vi "DropDetection NaamaVision.vi"(8 "error in":errorcluster, 10 "Minimum Match Score":sgl=400.0, 11 "Path":path=path "Z:/Downloads/Fridge Pictures/1") -> (0 "error out":errorcluster, 1 "Number of Matches":i32, 2 "Matches (pixel)":T1(array[cluster]), 3 "Image Out":T2(plugin-control))   [LabVIEW 2013]
uses:
  <vilib>/vision/NI_Vision_Development_Module.lvlib
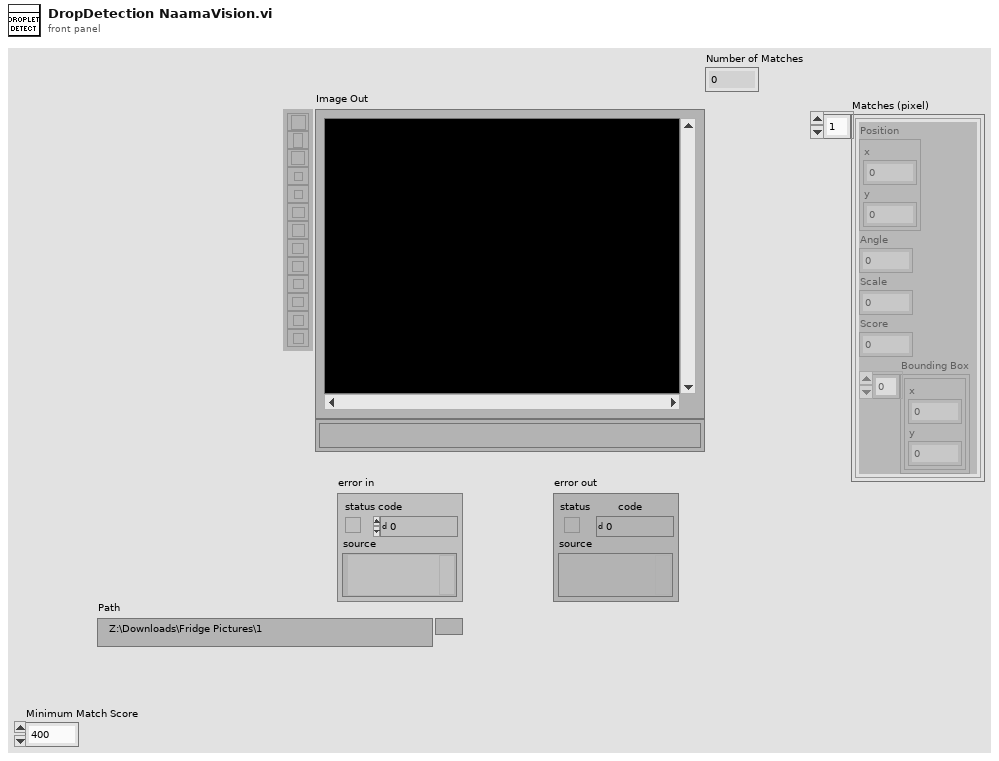
[diagram p1: front panel]
types:
  T1 = cluster{"Position":cluster{"x":sgl, "y":sgl}, "Angle":sgl, "Scale":sgl, "Score":sgl, "Bounding Box":cluster{"x":sgl, "y":sgl}[]}[]
  T2 = typedef "IMAQ Image.ctl" = refnum<image>
  T3 = cluster{"Global Rectangle":i32[], "Contours":cluster{"ID":enum32{"External", "Internal"}, "Type":u32, "Coordinates":i32[]}[]}
  T4 = typedef "Image Type" = u32
  T5 = cluster{"Number of Matches Requested":i32, "Minimum Match Score":sgl, "Angle Ranges":cluster{"Start Angle":sgl, "End Angle":sgl}[]}
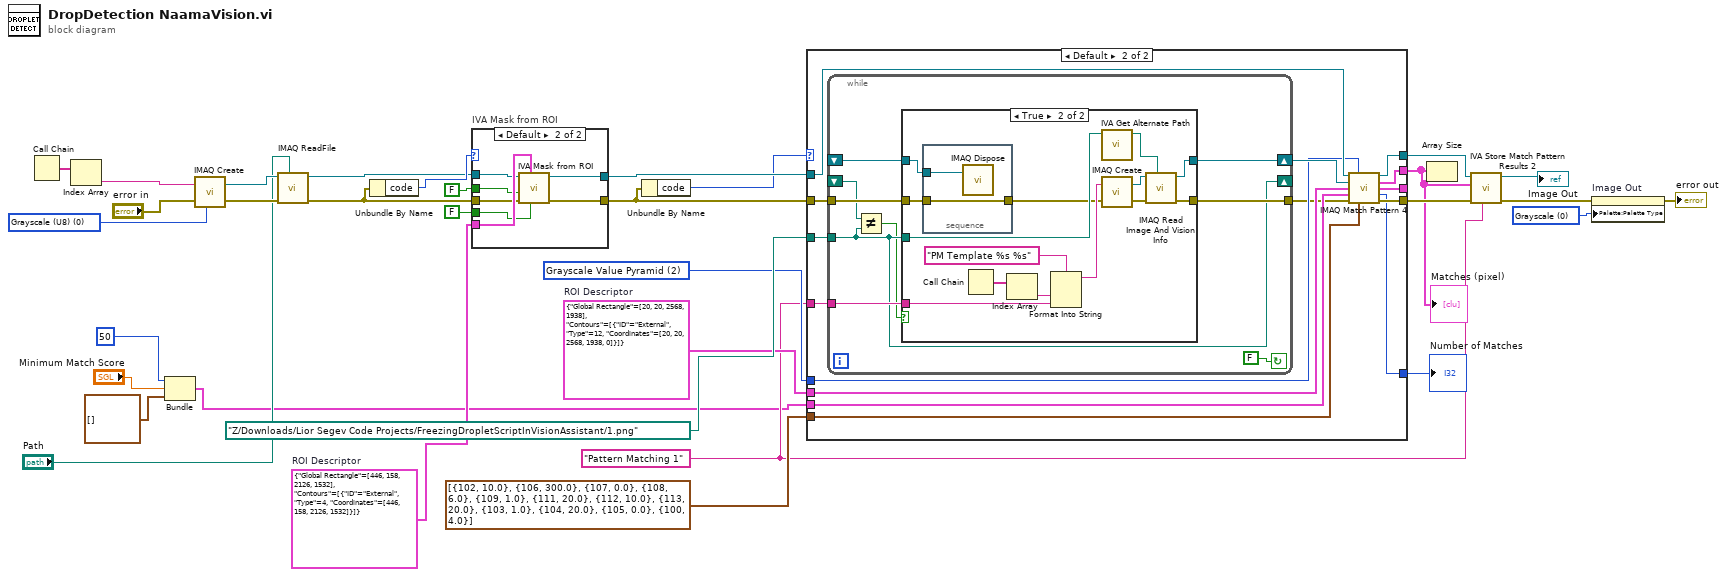
[diagram p0: block diagram]
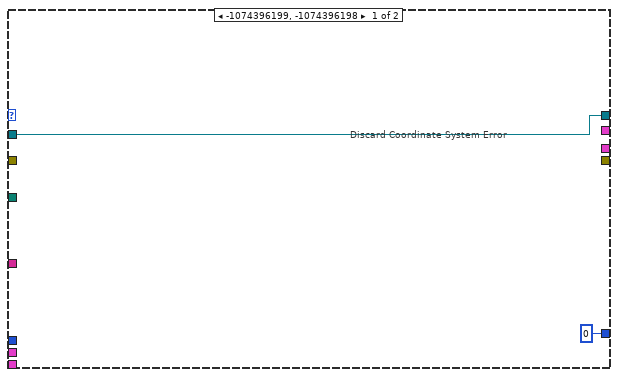
[diagram p2: hidden frame]
diagram:
  w11 = u32 0 items=["Grayscale", "Binary", "Gradient", "Rainbow", "Temperature", "User Defined"] ("Palette")
  w16 = 2 items=["All", "Low Discrepancy Sampling", "Grayscale Value Pyramid", "Gradients Pyramid"] ("Algorithm")
  w13 = "Pattern Matching 1" ("Step Name")
  w15 = T3 {"Global Rectangle"=[20, 20, 2568, 1938], "Contours"=[{"ID"=enum."External", "Type"=12, "Coordinates"=[20, 20, 2568, 1938, 0]}]}  # ROI Descriptor
  w27 = T3 {"Global Rectangle"=[446, 158, 2126, 1532], "Contours"=[{"ID"=enum."External", "Type"=4, "Coordinates"=[446, 158, 2126, 1532]}]}  # ROI Descriptor
  w28 = T4 0 items=["Grayscale (U8)", "Grayscale (I16)", "Grayscale (SGL)", "Complex (CSG)", "RGB (U32)", "HSL (U32)", "RGB (U64)", "Grayscale (U16)"] ("Image Type")
  n1 = Call Chain() -> (call chain=w30:string[])
  n2 = Index Array(array=w30) -> (element=w29:string)  [unwired: 1 in]
  n3 = Bundle("Number of Matches Requested"=50, "Minimum Match Score"="Minimum Match Score", "Angle Ranges"=cluster{"Start Angle":sgl, "End Angle":sgl}[] []) -> (w1:T5)  [unwired: 1 in]
  n4 = call "IMAQ Create"("Image Name"=w29, "Image Type"=w28, "error in (no error)"="error in") -> ("New Image"=w33:T2, "error out"=w32:errorcluster)  [unwired: 1 in, 1 out]
  n5 = call "IMAQ ReadFile"("File Path"="Path", "error in (no error)"=w32, "Image"=w33) -> ("error out"=w24:errorcluster, "Image Out"=w6:T2)  [unwired: 2 in, 5 out]
  n6 = Unbundle By Name(w24) -> ("code"=w23:i32)
  n7 = case "IVA Mask from ROI" shown="Default" w23 {
    tunnel: w27 -> [_ w41]
    tunnel: FALSE ("Shrink") -> [_ w40]
    tunnel: w6 -> [w34 w39]
    tunnel: w24 -> [_ w38]
    tunnel: [_ w37] -> w18
    tunnel: [w34 w36] -> w21
    tunnel: FALSE ("Out / In") -> [_ w35]
    frame -1074396199, -1074396198 {
      # "Discard\nCoordinate\nSystem\nError"
    }
    frame Default {
      n8 = call <vilib>:"IVA Mask from ROI.vi"("Shrink"=w40, "ROI Descriptor"=w41, "error in (no error)"=w38, "Out / In"=w35, "Image Src"=w39) -> ("error out"=w37:errorcluster, "Image Out"=w36:T2)  [unwired: 5 out]
    }
  }
  n9 = Unbundle By Name(w18) -> ("code"=w17:i32)
  n10 = case shown="Default" w17 {
    tunnel: path "Z:/Downloads/Lior Segev Code Projects/FreezingDropletScriptInVisionAssistant/1.png" ("Template File Path") -> [_ w58]
    tunnel: w18 -> [_ w57]
    tunnel: w21 -> [w43 w52]
    tunnel: [_ w53] -> w20
    tunnel: [_ w54] -> w12
    tunnel: [w43 w51] -> w19
    tunnel: w13 -> [_ w56]
    tunnel: w16 -> [_ w50]
    tunnel: w15 -> [_ w49]
    tunnel: w1 -> [_ w48]
    tunnel: cluster{"Item":u16, "Value":dbl}[] [{"Item"=102, "Value"=10.0}, {"Item"=106, "Value"=300.0}, {"Item"=107, "Value"=0.0}, {"Item"=108, "Value"=6.0}, {"Item"=109, "Value"=1.0}, {"Item"=111, "Value"=20.0}, {"Item"=112, "Value"=10.0}, {"Item"=113, "Value"=20.0}, {"Item"=103, "Value"=1.0}, {"Item"=104, "Value"=20.0}, {"Item"=105, "Value"=0.0}, {"Item"=100, "Value"=4.0}] ("Advanced Options") -> [_ w46]
    tunnel: [_ w45] -> _
    tunnel: [0 ("Number of Matches") w44] -> w7
    frame -1074396199, -1074396198 {
      # "Discard Coordinate System Error"
    }
    frame Default {
      n11 = while {
        shift-right: [w67] -> w55
        shift-left: _ -> [w66]
        tunnel: [w64] -> w47
        tunnel: w57 -> [w63]
        tunnel: w58 -> [w60]
        tunnel: w56 -> [w62]
        shift-right: [w60] -> _
        shift-left: _ -> [w61]
        stop <- FALSE continue-if-true
        n12 = Not Equal?(x=w61, y=w60) -> (x != y?=w59:bool)
        n13 = case shown="True" w59 {
          tunnel: [w69 w81] -> w67
          tunnel: w66 -> [w69 w72]
          tunnel: [w68 w78] -> w64
          tunnel: w63 -> [w68 w71]
          tunnel: w60 -> [_ w74]
          tunnel: w62 -> [_ w75]
          frame False {
          }
          frame True {
            n14 = stacked-sequence {
              tunnel: w72 -> [w85]
              tunnel: w71 -> [w84]
              tunnel: [w84] -> w70
              frame #0 {
                n15 = call "IMAQ Dispose"("Image"=w85) -> ()  [unwired: 2 in, 4 out]
              }
            }
            n16 = Call Chain() -> (call chain=w77:string[])
            n17 = Index Array(array=w77) -> (element=w76:string)  [unwired: 1 in]
            n18 = Format Into String(format string="PM Template %s %s" ("Image Name"), w76, w75) -> (resulting string=w83:string)  [unwired: 2 in, 1 out]
            n19 = call <vilib>:"IVA Get Alternate Path.vi"("Path In"=w74) -> ("Path Out"=w73:path)  [unwired: 10 out]
            n20 = call "IMAQ Create"("Image Name"=w83, "error in (no error)"=w70) -> ("New Image"=w80:T2, "error out"=w79:errorcluster)  [unwired: 2 in, 1 out]
            n21 = call "IMAQ Read Image And Vision Info"("File Path"=w73, "error in (no error)"=w79, "Image"=w80) -> ("error out"=w78:errorcluster, "Image Out"=w81:T2)  [unwired: 1 in, 6 out]
          }
        }
      }
      n22 = call "IMAQ Match Pattern 4"("Image"=w52, "Algorithm"=w50, "Template Image"=w55, "ROI Descriptor"=w49, "Parameters"=w48, "error in (no error)"=w47, "Advanced Options"=w46) -> ("Image (duplicate)"=w51:T2, "Matches (pixel)"=w54:T1, "Matches (real-world)"=w45:T1, "Number of Matches"=w44:i32, "error out"=w53:errorcluster)  [unwired: 4 in]
    }
  }
  "Matches (pixel)" <- w12
  "Number of Matches" <- w7
  n23 = Array Size(array=w12) -> ()  [unwired: 1 out]
  n24 = call <vilib>:"IVA Store Match Pattern Results 2.vi"("Step Name"=w13, "error in (no error)"=w20, "Matches (pixel)"=w12, "Image in"=w19) -> ("error out"=w10:errorcluster, "Image dup"=→"Image Out":T2)  [unwired: 2 in, 4 out]
  n25 = property on="Image Out" class="ImageControl"(error in=w10, "Palette:Palette Type"=w11) -> (error out=→"error out":errorcluster)  [unwired: 1 in, 1 out]
